vi "Get Bus Controller and Remote Terminals Handles from BTI Channel.vi"(8 "error in":errorcluster, 10 "terminal addresses":T1[](array[typedef]), 11 "channel handle in":u64) -> (0 "error out":errorcluster, 1 "remote terminal handles out":u64[](array[numeric]), 2 "bus controller handle out":u64, 3 "channel handle out":u64)   [LabVIEW 2020, in "AIM MIL-STD-1553 Engine.lvlib" / "Implementation.lvlib" / "Tx Acyclic Execution Unit.lvclass"]
uses:
  Tx Acyclic Execution Unit.lvclass
  <instrlib>/BTI1553Lib/BTI1553LV.lvlib
  Shared/Address.ctl
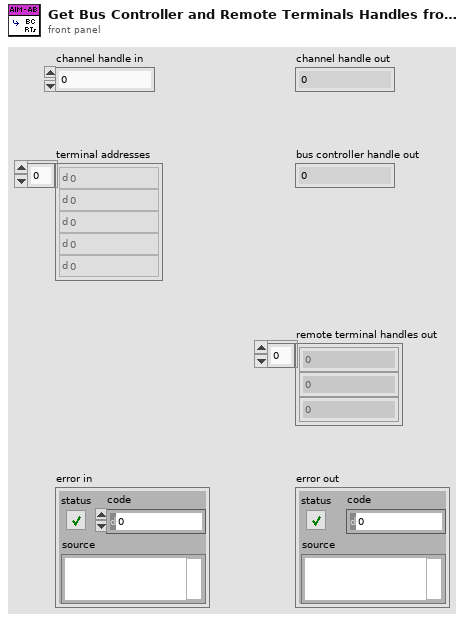
[diagram p1: front panel]
types:
  T1 = typedef "Address.ctl" = u16
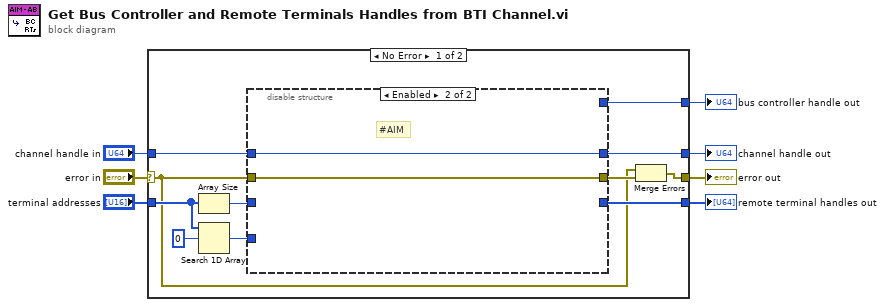
[diagram p0: block diagram]
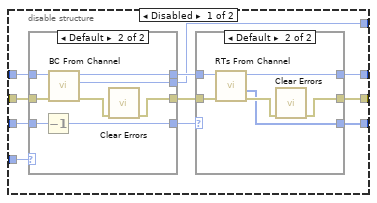
[diagram p2: hidden frame]
diagram:
  n1 = case shown="No Error" "error in" {
    selector: "error in" -> [w8 w51]
    tunnel: "channel handle in" -> [w18 w52]
    tunnel: [w9 w51] -> w5
    tunnel: [w17 w52] -> w4
    tunnel: "terminal addresses" -> [w13 _]
    tunnel: [w14 _] -> w2
    tunnel: [w10 _] -> w1
    frame No Error {
      n2 = Array Size(array=w13) -> (size(s)=w12:i32)
      n3 = Search 1D Array(1D array=w13, element=T1 0) -> (index of element=w15:i32)  [unwired: 1 in]
      n4 = disable-structure shown="Enabled" {
        disable-tunnel: w18 -> [w28 w50]
        disable-tunnel: [w27 w50] -> w17
        disable-tunnel: w15 -> [w26 _]
        disable-tunnel: [w25 _] -> w14
        disable-tunnel: w12 -> [w24 _]
        disable-tunnel: [w22 w49] -> w11
        disable-tunnel: [w20 _] -> w10
        disable-tunnel: w8 -> [w19 w49]
        frame Disabled {
          n5 = case shown="Default" w26 {
            tunnel: [w40 w48] -> w29
            tunnel: w28 -> [w40 w47]
            tunnel: w19 -> [w39 w46]
            tunnel: [w39 w41] -> w21
            tunnel: [_ w44] -> w25
            tunnel: w24 -> [w38 w43]
            tunnel: [w38 w42] -> w23
            frame -1 {
            }
            frame Default {
              n6 = Decrement(x=w43) -> (x-1=w42:i32)
              n7 = call <instrlib>:"BC From Channel.vi"("error in (no error)"=w46, "channel handle in"=w47) -> ("error out"=w45:errorcluster, "bus controller handle out"=w44:u64, "channel handle out"=w48:u64)  [unwired: 7 in]
              n8 = call <vilib>:"Clear Errors.vi"("error in (no error)"=w45) -> ("error out"=w41:errorcluster)  [unwired: 5 in, 1 out]
            }
          }
          n9 = case shown="Default" w23 {
            tunnel: w29 -> [w31 w37]
            tunnel: [w31 w36] -> w27
            tunnel: [w30 w32] -> w22
            tunnel: w21 -> [w30 w35]
            tunnel: [_ w33] -> w20
            frame ..0 {
            }
            frame Default {
              n10 = call <instrlib>:"RTs From Channel.vi"("error in (no error)"=w35, "channel handle in"=w37) -> ("error out"=w34:errorcluster, "remote terminal handles out"=w33:u64[], "channel handle out"=w36:u64)  [unwired: 6 in, 1 out]
              n11 = call <vilib>:"Clear Errors.vi"("error in (no error)"=w34) -> ("error out"=w32:errorcluster)  [unwired: 5 in, 1 out]
            }
          }
        }
        frame Enabled {
          # "#AIM"
        }
      }
      n12 = Merge Errors(w8, w11) -> (w9:errorcluster)
    }
    frame Error {
    }
  }
  "bus controller handle out" <- w2
  "remote terminal handles out" <- w1
  "error out" <- w5
  "channel handle out" <- w4
